vi "prepareSharedVariables.vi"(8 "error in (no error)":errorcluster, 11 "DataListenerThisComponent in":refnum<class "DataListenerThisComponent.lvclass">) -> (0 "error out":errorcluster, 3 "DataListenerThisComponent out":refnum<class "DataListenerThisComponent.lvclass">)   [LabVIEW 2015]
uses:
  ComponentTemplateCore/ComponentModel/ComponentModelDT/ConfigurationFileReaderDT/ConfigurationFileReaderDT.lvclass
  ComponentTemplateCore/ComponentModel/ComponentModel/Typedefs/CommunicationConfig.ctl
  ComponentTemplateCore/ComponentModel/ComponentModel/Typedefs/SVProcessConfig.ctl
  DataListenerThisComponent.lvclass
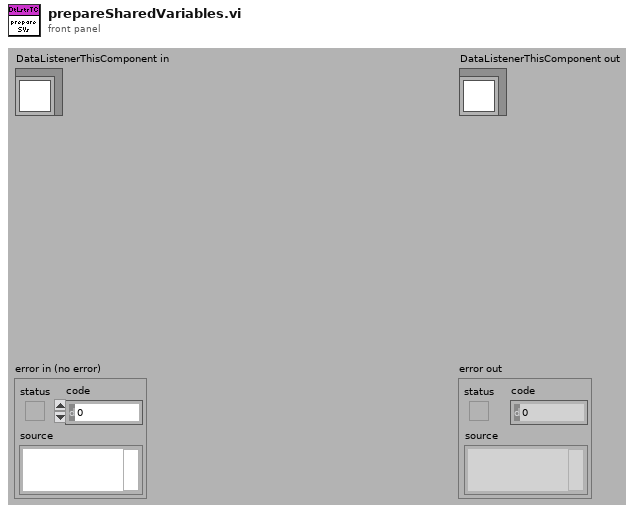
[diagram p1: front panel]
types:
  T1 = typedef "SVProcessConfig.ctl" = cluster{"subDataProcessPrototype":string, "pubDataProcessPrototype":string, "commandProcessPrototype":string, "commandSVName":string}
  T2 = typedef "CommunicationConfig.ctl" = cluster{"hostComputerAddress":string, "ComponentAcronym":string, "InstanceIdentifier":i32}
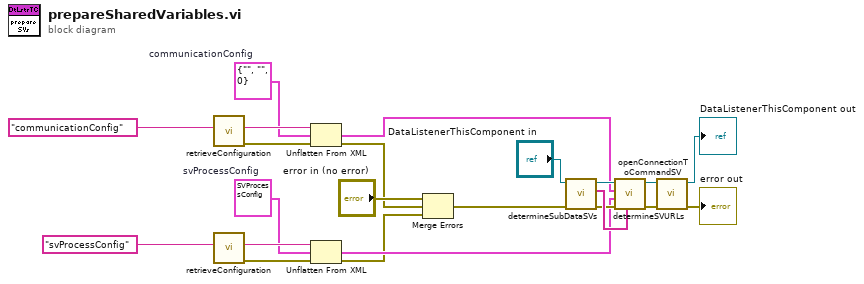
[diagram p0: block diagram]
diagram:
  w15 = T1 {"subDataProcessPrototype"="SubDataSV", "pubDataProcessPrototype"="PubDataSV", "commandProcessPrototype"="CommandSV", "commandSVName"="Command"}  # svProcessConfig
  w19 = T2 {"hostComputerAddress"="", "ComponentAcronym"="", "InstanceIdentifier"=0}  # communicationConfig
  n1 = call "retrieveConfiguration.vi"("dataName"="communicationConfig") -> ("error out"=w20:errorcluster, "dataValueFromFile"=w21:string)  [unwired: 8 in, 1 out]
  n2 = call "retrieveConfiguration.vi"("dataName"="svProcessConfig") -> ("error out"=w18:errorcluster, "dataValueFromFile"=w17:string)  [unwired: 8 in, 1 out]
  n3 = Unflatten From XML(xml string=w21, type=w19, error in (no error)=w20) -> (value=w7:T2, error out=w3:errorcluster)
  n4 = Unflatten From XML(xml string=w17, type=w15, error in (no error)=w18) -> (value=w6:T1, error out=w2:errorcluster)
  n5 = Merge Errors("error in (no error)", w3, w2) -> (w1:errorcluster)
  n6 = call "determineSubDataSVs.vi"("error in (no error)"=w1, "DataListenerThisComponent in"="DataListenerThisComponent in") -> ("error out"=w8:errorcluster, "svNames"=w12:string[], "DataListenerThisComponent out"=w10:refnum<class "DataListenerThisComponent.lvclass">)  [unwired: 7 in]
  n7 = call-dynamic "determineSVURLs.vi"("SVNames"=w12, "error in (no error)"=w8, "svProcessConfig"=w6, "communicationConfig"=w7, "DataListener in"=w10) -> ("error out"=w13:errorcluster, "DataListener out"=w14:refnum<class "DataListenerThisComponent.lvclass">)  [unwired: 5 in]
  n8 = call-dynamic "openConnectionToCommandSV.vi"("error in (no error)"=w13, "DataListener in"=w14) -> ("error out"=→"error out":errorcluster, "DataListener out"=→"DataListenerThisComponent out":refnum<class "DataListenerThisComponent.lvclass">)  [unwired: 8 in]
